vi "mergemain.vi"   [LabVIEW 2013]
uses:
  arguments.ctl
  kernel32.dll
types:
  T1 = typedef "arguments.ctl" = cluster{"working directory":string, "flags":string[], "values":string[]}
  T2 = enum32{"invalid app kind", "Development System", "Run Time System", "Student Edition", "Embedded LabVIEW", "Evaluation", "Custom"}
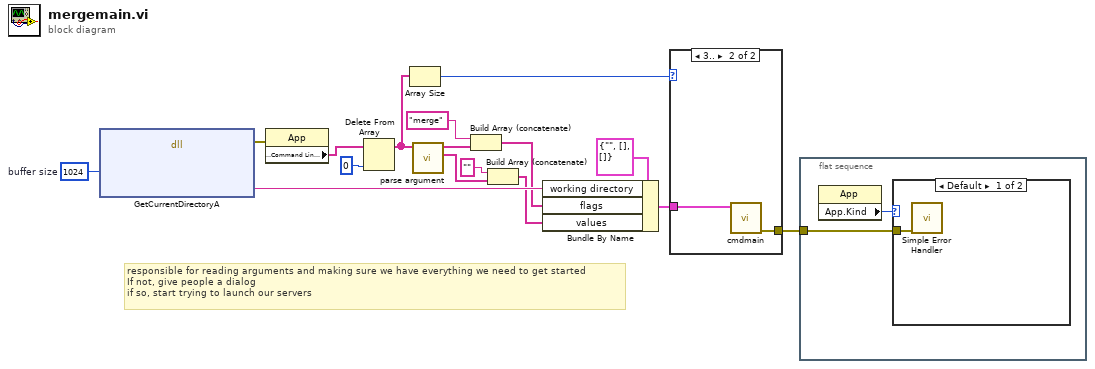
[diagram p0: block diagram]
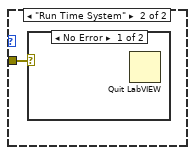
[diagram p2: hidden frame]
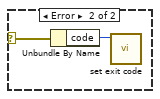
[diagram p3: hidden frame]
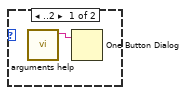
[diagram p4: hidden frame]
diagram:
  w15 = 1024  # buffer size
  # "responsible for reading arguments and making sure we have everything we need to get started\nIf not, give people a dialog\nif so, start trying to launch our servers"
  n1 = dll-call lib="kernel32.dll" fn="GetCurrentDirectoryA" ("Kernel32.dll - \nGetCurrentDirectoryA")("nBufferLength"=w15) -> (error out=w13:errorcluster, "lpBuffer"=w9:string)  [unwired: 5 in, 2 out]
  n2 = property class="App"(error in=w13) -> ("Application:Command Line Arguments"=w16:string[])  [unwired: 1 in, 2 out]
  n3 = Delete From Array(array=w16, index=0) -> (array with subset deleted=w11:string[])  [unwired: 1 in, 1 out]
  n4 = Array Size(array=w11) -> (size(s)=w1:i32)
  n5 = call "parse argument.vi"("Arguments"=w11) -> ("values"=w3:string[], "flags"=w7:string[])  [unwired: 9 in]
  n6 = Build Array (concatenate)("merge", w7) -> (w6:string[])
  n7 = Build Array (concatenate)("", w3) -> (w2:string[])
  n8 = Bundle By Name(cluster=T1 {"working directory"="", "flags"=[], "values"=[]} ("command line arguments"), "working directory"=w9, "flags"=w6, "values"=w2) -> (w8:T1)
  n9 = case shown="3.." w1 {
    tunnel: [_ w19] -> w12
    tunnel: w8 -> [_ w18]
    frame ..2 {
      n10 = call "arguments help.vi"() -> ("args help"=w17:string)  [unwired: 11 in]
      n11 = One Button Dialog(message=w17) -> ()  [unwired: 1 in, 1 out]
    }
    frame 3.. {
      n12 = call "cmdmain.vi"("command line arguments"=w18) -> ("error out"=w19:errorcluster)  [unwired: 10 in]
    }
  }
  n13 = flat-sequence {
    tunnel: w12 -> [w21]
    frame #0 {
      n14 = property class="App"() -> ("App.Kind"=w20:T2)  [unwired: 2 in, 2 out]
      n15 = case shown="Default" w20 {
        tunnel: w21 -> [w22 w23]
        frame Default {
          n16 = call <vilib>:"Simple Error Handler.vi"("error in (no error)"=w22) -> ()  [unwired: 4 in, 5 out]
        }
        frame "Run Time System" {
          n17 = case shown="No Error" w23 {
            selector: w23 -> [_ w25]
            frame No Error {
              n18 = Quit LabVIEW() -> ()  [unwired: 1 in]
            }
            frame Error {
              n19 = Unbundle By Name(w25) -> ("code"=w24:i32)
              n20 = call "set exit code.vi"("exit code"=w24) -> ()  [unwired: 11 in]
            }
          }
        }
      }
    }
  }
